vi "4_5a.vi"() -> ()   [LabVIEW 2020]
panel:
  out "Output1":string
  out "Output2":string
  in  "Word":string
  in  "Input":string
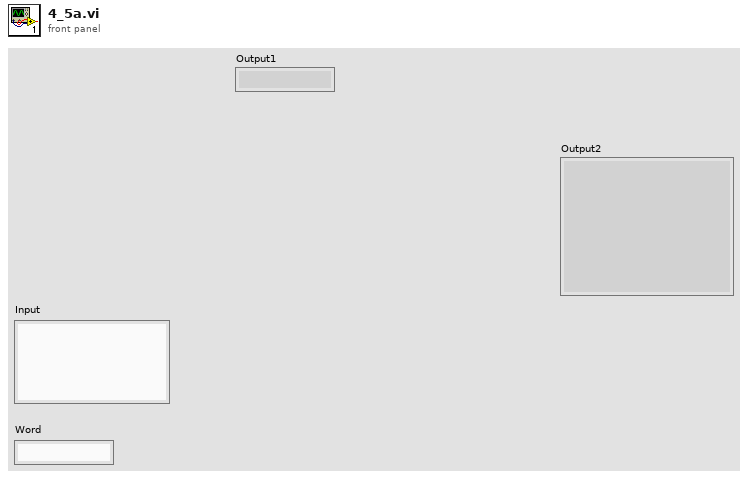
[diagram p1: front panel]
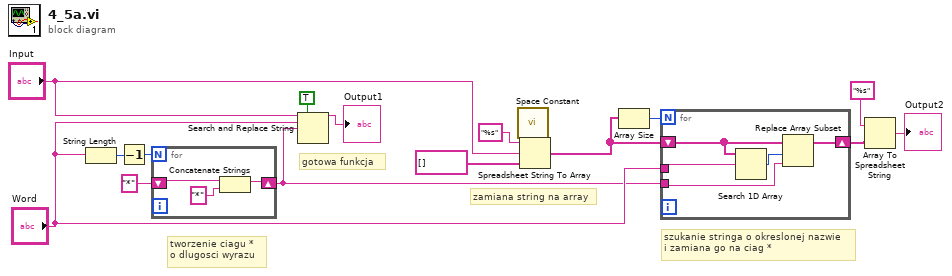
[diagram p0: block diagram]
diagram:
  # "szukanie stringa o okreslonej nazwie\ni zamiana go na ciag *"
  # "zamiana string na array"
  # "gotowa funkcja"
  # "tworzenie ciagu * \no dlugosci wyrazu"
  n1 = String Length(string="Word") -> (length=w15:i32)
  n2 = Decrement(x=w15) -> (x-1=w13:i32)
  n3 = for {
    N: w13 -> [_]
    shift-right: [w17] -> w5
    shift-left: "*" -> [w19]
    n4 = Concatenate Strings(w19, "*" ("replace string (\"\")")) -> (w17:string)
  }
  n5 = Search and Replace String(replace all?=TRUE, input string="Input", search string="Word", replace string=w5) -> (result string=→"Output1":string)  [unwired: 4 in, 3 out]
  n6 = call <vilib>:"Space Constant.vi"() -> ("String"=w10:string)
  n7 = Spreadsheet String To Array(delimiter (Tab)=w10, format string="%s", spreadsheet string="Input", array type (2D Dbl)=string[] []) -> (array=w7:string[])
  n8 = Array Size(array=w7) -> (size(s)=w8:i32)
  n9 = for {
    N: w8 -> [_]
    tunnel: "Word" -> [w24]
    tunnel: w5 -> [w21]
    shift-right: [w20] -> w4
    shift-left: w7 -> [w23]
    n10 = Search 1D Array(1D array=w23, element=w24) -> (index of element=w22:i32)  [unwired: 1 in]
    n11 = Replace Array Subset(array=w23, new element=w21, index=w22) -> (w20:string[])
  }
  n12 = Array To Spreadsheet String(array=w4, 3:"%s") -> (spreadsheet string=→"Output2":string)  [unwired: 1 in]
